vi "Manual_Level_Shift.vi"() -> ()   [LabVIEW 2014]
panel:
  in  "cluster":cluster{}
  in  "Down":bool=TRUE
  in  "Up":bool=TRUE
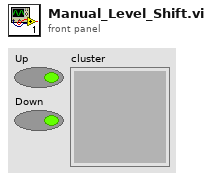
[diagram p1: front panel]
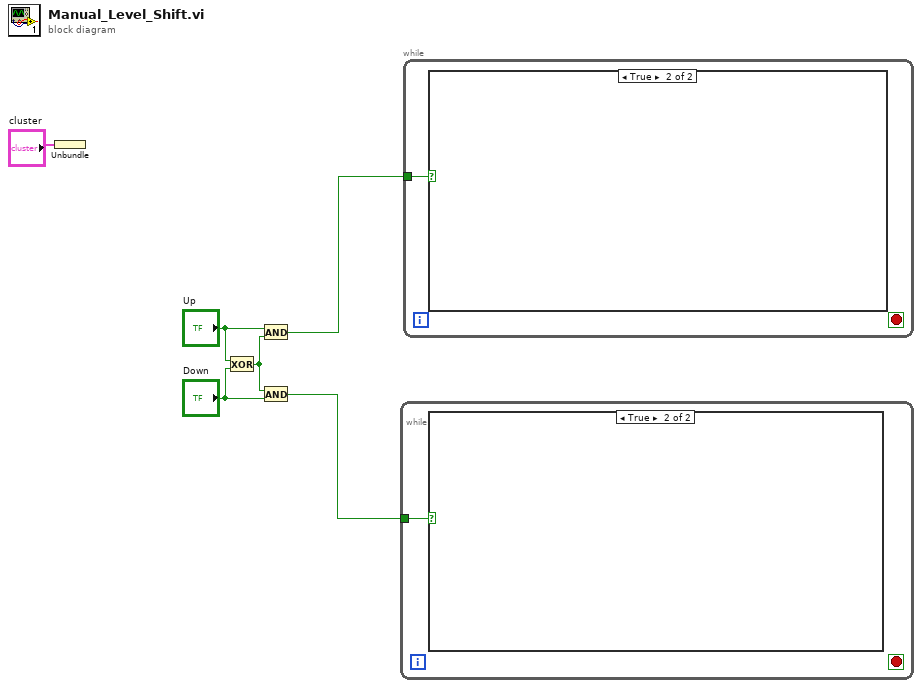
[diagram p0: block diagram]
diagram:
  n1 = Unbundle("cluster") -> ()  [unwired: 1 out]
  n2 = Exclusive Or(1:"Down", 2:"Up") -> (0:w6:bool)
  n3 = And(x="Up", y=w6) -> (x .and. y?=w3:bool)
  n4 = And(x=w6, y="Down") -> (x .and. y?=w2:bool)
  n5 = while {
    tunnel: w2 -> [w7]
    stop <- _ stop-if-true
    n6 = case shown="True" w7 {
      frame False {
      }
      frame True {
      }
    }
  }
  n7 = while {
    tunnel: w3 -> [w8]
    stop <- _ stop-if-true
    n8 = case shown="True" w8 {
      frame False {
      }
      frame True {
      }
    }
  }
